vi "VI Server_Table_UpdatItemList.vi"(6 "New Value":string[][](table), 7 "Label":string, 8 "error in":errorcluster, 11 "VI Server Cluster":T1) -> (0 "error out":errorcluster, 1 "Table.Ref":refnum<vi>, 3 "VI Server Cluster.DUP":T1)   [LabVIEW 2020, in "VI Server Toolkit LV2013.lvlib"]
doc: "Updates Table content/value."
uses:
  VI Server Toolkit LV2013.lvlib
  VI Server_TypeDefs/VI Server_RefsCluster.ctl
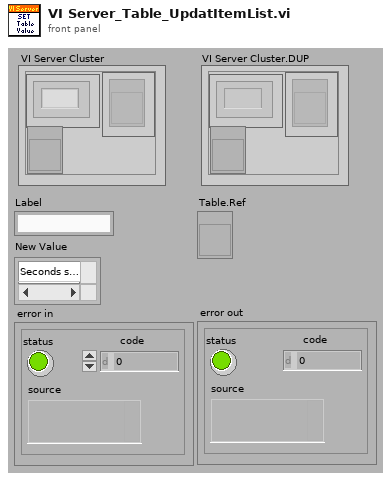
[diagram p1: front panel]
types:
  T1 = typedef "VI Server_RefsCluster.ctl" = cluster{"Labels":string[], "Refs":refnum<vi>[], "VI Ref":refnum<vi>}
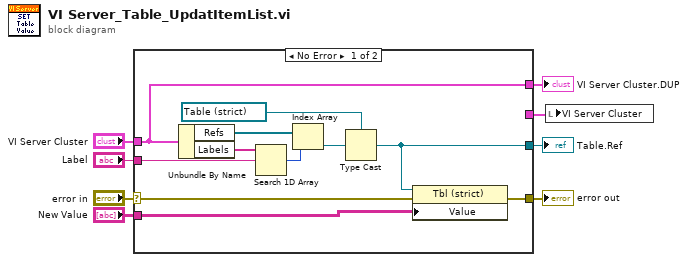
[diagram p0: block diagram]
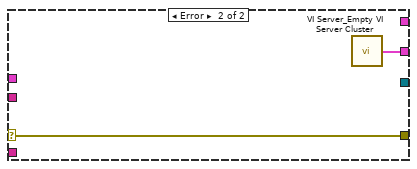
[diagram p2: hidden frame]
diagram:
  n1 = case shown="No Error" "error in" {
    selector: "error in" -> [w14 w21]
    tunnel: "Label" -> [w18 _]
    tunnel: "VI Server Cluster" -> [w10 _]
    tunnel: [w13 w21] -> w8
    tunnel: [w12 _] -> w3
    tunnel: "New Value" -> [w11 _]
    tunnel: [w10 _] -> w2
    tunnel: [_ w20] -> w1
    frame No Error {
      n2 = Unbundle By Name(w10) -> ("Refs"=w16:refnum<vi>[], "Labels"=w19:string[])
      n3 = Search 1D Array(1D array=w19, element=w18) -> (index of element=w17:i32)  [unwired: 1 out]
      n4 = Index Array(array=w16, index=w17) -> (element=w15:refnum<vi>)
      n5 = Type Cast(type=refnum<vi> refnum ("Table"), x=w15) -> (*(type *) &x=w12:refnum<vi>)
      n6 = property class="Tbl (strict)"(reference=w12, error in=w14, "Value"=w11) -> (error out=w13:errorcluster)  [unwired: 1 out]
    }
    frame Error {
      n7 = call "VI Server_Empty VI Server Cluster.vi"() -> ("VI Server Cluster"=w20:T1)  [unwired: 7 in]
    }
  }
  "error out" <- w8
  "VI Server Cluster.DUP" <- w2
  "Table.Ref" <- w3
  n8 = local write "VI Server Cluster"(w1) -> ()
